vi "Custom Send.vi"(1 "Command In":string) -> (0 "Command Out":string)   [LabVIEW 2017]
panel:
  in  "VBUS":u8=1 max=1
  in  "BATC":u8=3 max=3
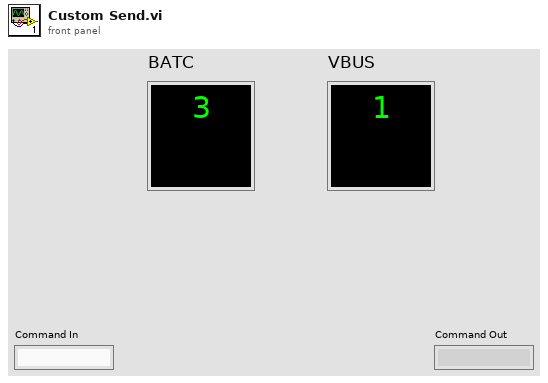
[diagram p1: front panel]
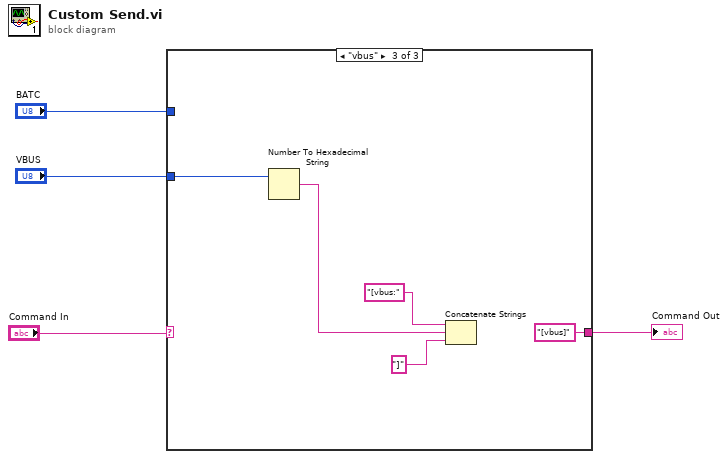
[diagram p0: block diagram]
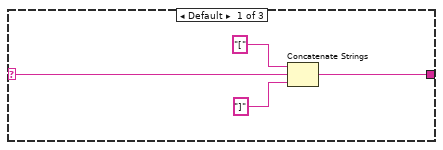
[diagram p2: hidden frame]
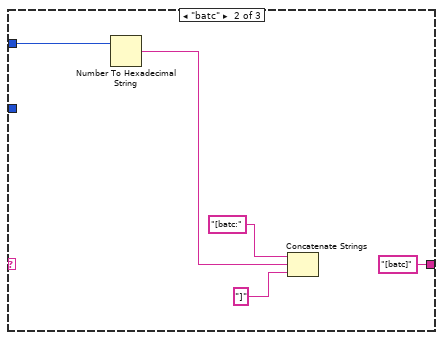
[diagram p3: hidden frame]
diagram:
  n1 = case shown="\"vbus\"" "Command In" {
    selector: "Command In" -> [w8 _ _]
    tunnel: "BATC" -> [_ w13 _]
    tunnel: "VBUS" -> [_ _ w15]
    tunnel: [w7 "[batc]" "[vbus]"] -> w1
    frame Default {
      n2 = Concatenate Strings("[" ("string"), w8, "]" ("string")) -> (w7:string)
    }
    frame "batc" {
      n3 = Number To Hexadecimal String(2:w13) -> (0:w12:string)  [unwired: 1 in]
      n4 = Concatenate Strings("[batc:" ("string"), w12, "]" ("string")) -> ()  [unwired: 1 out]
    }
    frame "vbus" {
      n5 = Number To Hexadecimal String(2:w15) -> (0:w17:string)  [unwired: 1 in]
      n6 = Concatenate Strings("[vbus:" ("string"), w17, "]" ("string")) -> ()  [unwired: 1 out]
    }
  }
  "Command Out" <- w1
